vi "blokada wysylania jazda.vi"(6 "wysylanie":bool, 10 "X axis":i32, 11 "Y axis":i32) -> (0 "fall edge wysl":bool, 1 "zak1":bool, 2 "zak2":bool, 3 "blokada jazdy":bool)   [LabVIEW 2015]
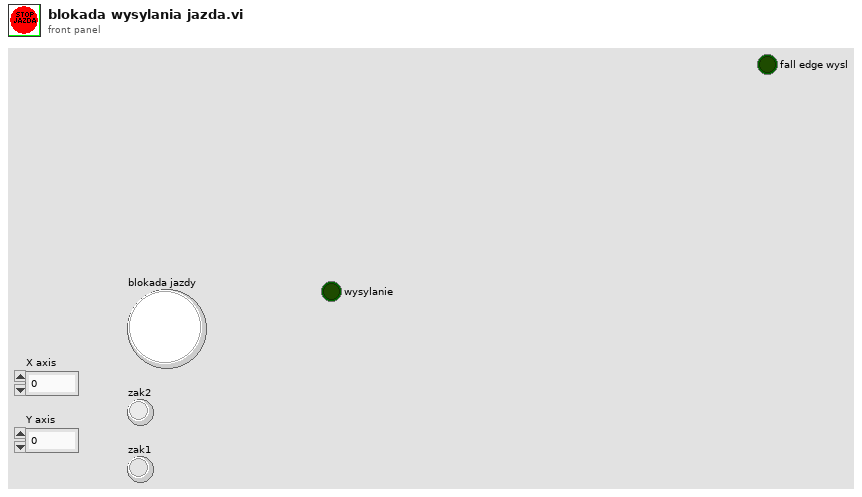
[diagram p1: front panel]
types:
  T1 = enum16{"Rising Edge", "Falling Edge", "Any Edge"}
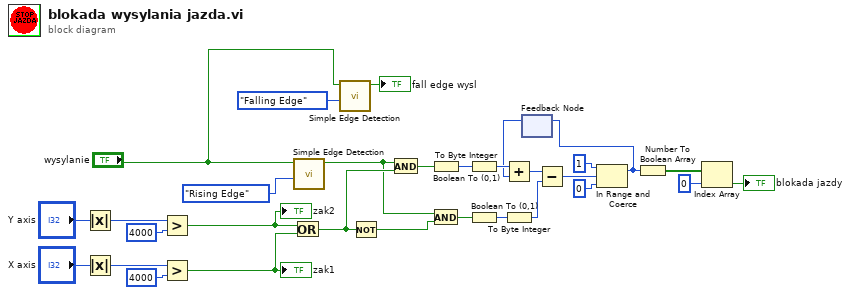
[diagram p0: block diagram]
diagram:
  n1 = Absolute Value(x="Y axis") -> (abs(x)=w21:i32)
  n2 = Absolute Value(x="X axis") -> (abs(x)=w24:i32)
  n3 = Greater?(x=w21, y=4000) -> (0:w29:bool)
  "zak2" <- w29
  n4 = Greater?(x=w24, y=4000) -> (0:w30:bool)
  "zak1" <- w30
  n5 = Or(x=w29, y=w30) -> (x .or. y?=w28:bool)
  n6 = call "Simple Edge Detection.vi"("Mode"=T1."Rising Edge", "clk_in"="wysylanie") -> ("edge?"=w5:bool)  [unwired: 9 in]
  n7 = call "Simple Edge Detection.vi"("Mode"=T1."Falling Edge", "clk_in"="wysylanie") -> ("edge?"=→"fall edge wysl":bool)  [unwired: 9 in]
  n8 = Not(x=w28) -> (.not. x?=w27:bool)
  n9 = And(x=w5, y=w28) -> (x .and. y?=w19:bool)
  n10 = Boolean To (0,1)(Boolean=w19) -> (0, 1=w11:i16)
  n11 = And(x=w5, y=w27) -> (x .and. y?=w20:bool)
  n12 = To Byte Integer(number=w11) -> (8bit integer=w10:i8)
  n13 = Boolean To (0,1)(Boolean=w20) -> (0, 1=w9:i16)
  n14 = To Byte Integer(number=w9) -> (8bit integer=w8:i8)
  n15 = feedback #1() -> (w6:i8)  [unwired: 1 in]
  n16 = Add(x=w10, y=w6) -> (x+y=w18:i8)
  n17 = Subtract(x=w18, y=w8) -> (x-y=w17:i8)
  n18 = In Range and Coerce(upper limit=i8 1 ("lower limit"), x=w17, lower limit=i8 0) -> (coerced(x)=w7:i8)  [unwired: 1 out]
  n19 = feedback-in #1(w7) -> ()
  n20 = Number To Boolean Array(number=w7) -> (Boolean array=w13:bool[])
  n21 = Index Array(array=w13, index=0) -> (element=→"blokada jazdy":bool)
